vi "Get Error Info.vi"(8 "Error In":errorcluster) -> (0 "Error Out":errorcluster, 4 "Time Stamp":timestamp, 5 "Error Name":string, 6 "Error Source":string, 7 "Error Scope":string)   [LabVIEW 2016, in "Stream Error.lvlib"]
doc: "--\nCopyright © 2017 Composed SystemsI All rights reserved.\n\nAuthor: Jon McBee <jon.mcbee@composed.io>\n\nThis library is provided \"AS IS\" ,WITHOUT WARRANTIES OR\nCONDITIONS OF ANY KIND, either express or implied.\n\nComposed Systems -- composed.io\n\nStream 0.0.1.1\nJon McBee - Composed Systems\nCopyright (c) 2017, Composed Systems"
uses:
  <userlib>/Composed Systems/Stream/Error/Stream Error.lvlib
  <userlib>/Composed Systems/Stream/Error/Classes/Error Interface/Error UID.ctl
  <userlib>/Composed Systems/Stream/Error/Classes/Error Interface/Error Interface.lvclass
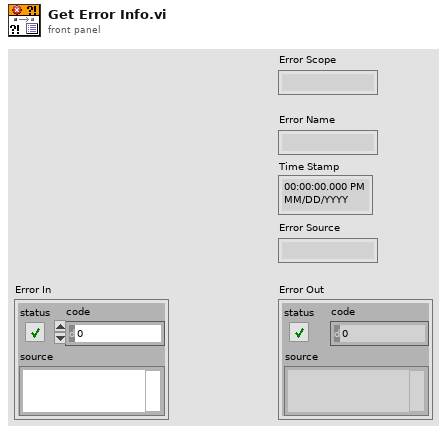
[diagram p1: front panel]
types:
  T1 = typedef "Stream Error.lvlib/Error Interface.lvclass/Error UID.ctl" = u16
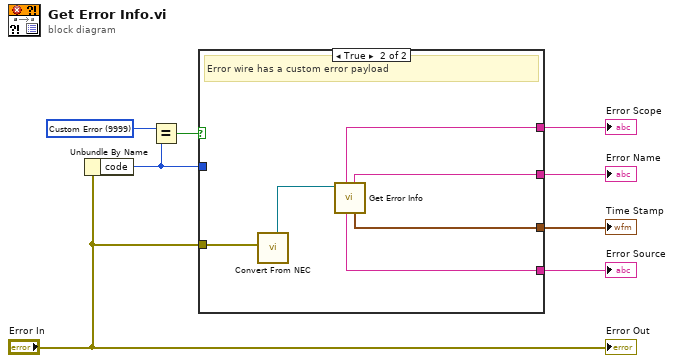
[diagram p0: block diagram]
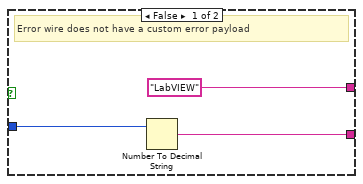
[diagram p2: hidden frame]
diagram:
  w4 = T1 9999 items=["Custom Error"=9999] ("Custom Error Codes")
  n1 = Unbundle By Name("Error In") -> ("code"=w7:i32)
  n2 = Equal?(x=w4, y=w7) -> (x = y?=w8:bool)
  n3 = case shown="True" w8 {
    tunnel: w7 -> [w11 _]
    tunnel: [w10 w15] -> w6
    tunnel: ["LabVIEW" w14] -> w5
    tunnel: "Error In" -> [_ w17]
    tunnel: [_ w13] -> w2
    tunnel: [_ w12] -> w1
    frame False {
      # "Error wire does not have a custom error payload"
      n4 = Number To Decimal String(number=w11) -> (decimal integer string=w10:string)  [unwired: 1 in]
    }
    frame True {
      # "Error wire has a custom error payload"
      n5 = call <userlib>:"Convert From NEC.vi"("error in (no error)"=w17) -> ("Error Interface out"=w16:refnum<class "Error Interface.lvclass">)  [unwired: 9 in, 1 out]
      n6 = call-dynamic "Get Error Info.vi"("Error Interface in"=w16) -> ("Time Stamp"=w12:timestamp, "Error Name"=w15:string, "Error Source"=w13:string, "Error Scope"=w14:string)  [unwired: 6 in, 1 out]
    }
  }
  "Error Scope" <- w5
  "Error Name" <- w6
  "Error Source" <- w2
  "Time Stamp" <- w1
  "Error Out" <- "Error In"
